vi "Digital Input Signals.vi"(8 "error in (no error)":errorcluster, 10 "Digital Input Signals":digitalwaveform[](array[waveform]), 11 "Digital Input Interface Messages in":refnum<class "Digital Input Interface Messages.lvclass">) -> (0 "error out":errorcluster, 3 "Digital Input Interface Messages out":refnum<class "Digital Input Interface Messages.lvclass">)   [LabVIEW 2021, in "Digital Input Interface Messages.lvlib" / "Digital Input Interface Messages.lvclass"]
uses:
  Digital Input Interface Messages.lvclass
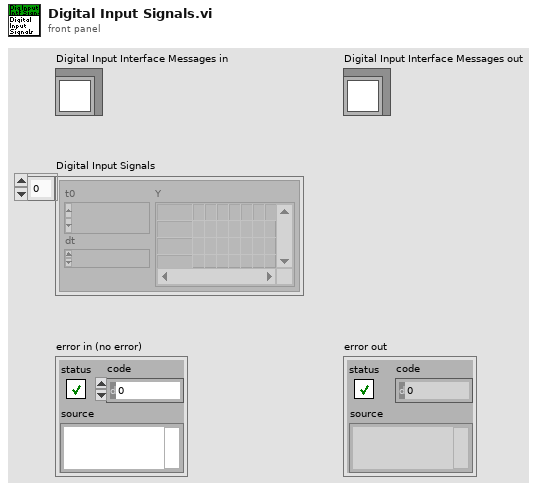
[diagram p1: front panel]
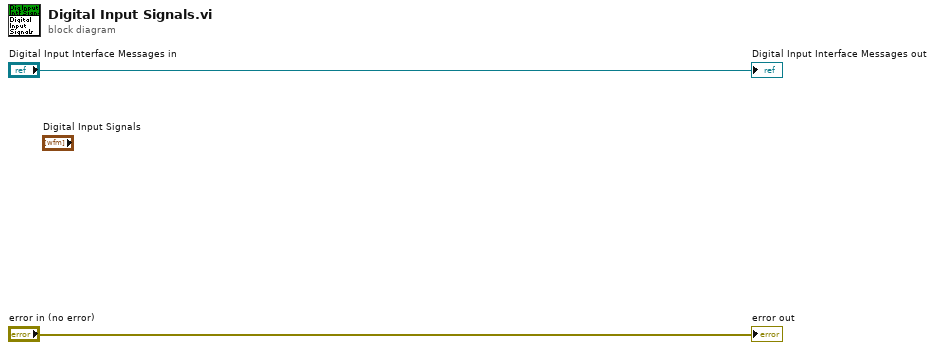
[diagram p0: block diagram]
diagram:
  "error out" <- "error in (no error)"
  "Digital Input Interface Messages out" <- "Digital Input Interface Messages in"
